vi "log queue.vi"(7 "action (get)":enum16{"init", "get", "close"}(ring)=enum."get") -> (3 "queue out":refnum<queue>)   [LabVIEW 2019]
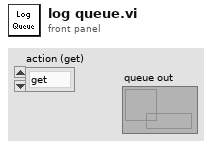
[diagram p1: front panel]
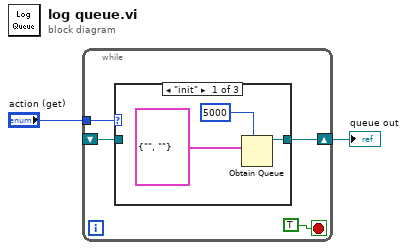
[diagram p0: block diagram]
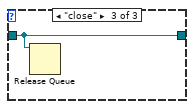
[diagram p3: hidden frame]
diagram:
  n1 = while {
    tunnel: "action (get)" -> [w5]
    shift-right: [w4] -> w1
    shift-left: _ -> [w3]
    stop <- TRUE stop-if-true
    n2 = case shown="\"init\"" w5 {
      tunnel: [w7 w10 w11] -> w4
      tunnel: w3 -> [_ w10 w11]
      frame "init" {
        n3 = Obtain Queue(max queue size (-1, unlimited)=5000, element data type=cluster{"time":string, "message":string} {"time"="", "message"=""}) -> (queue out=w7:refnum<queue>)  [unwired: 3 in, 2 out]
      }
      frame "get", Default {
      }
      frame "close" {
        n4 = Release Queue(queue=w11) -> ()  [unwired: 2 in, 3 out]
      }
    }
  }
  "queue out" <- w1
